vi "Write Map DVR 2.vi"(8 "error in (no error)":errorcluster, 10 "Map DVR":T1, 11 "Awesome! in":refnum<class "Awesome!.lvclass">) -> (0 "error out":errorcluster, 3 "Awesome! out":refnum<class "Awesome!.lvclass">)   [LabVIEW 2016, in "Awesome!.lvclass"]
uses:
  Awesome!.lvclass
  Common/Map DVR.ctl
  Common/Location Data.ctl
  Awesome!.lvclass/Awesome!.ctl
  Common/Common.lvlib
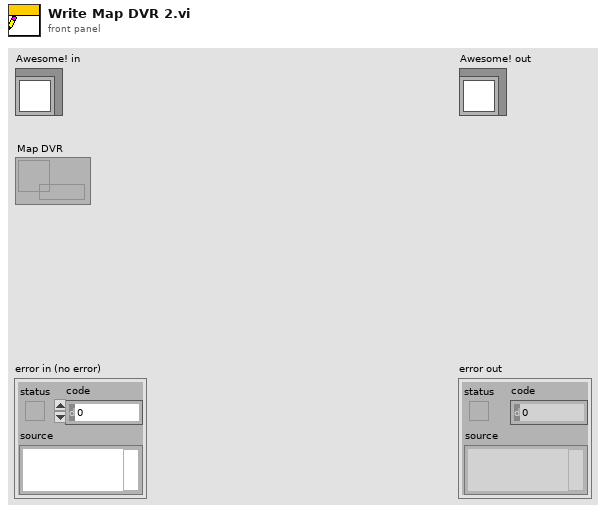
[diagram p1: front panel]
types:
  T1 = typedef "Common.lvlib/Map DVR.ctl" = refnum<data-value>
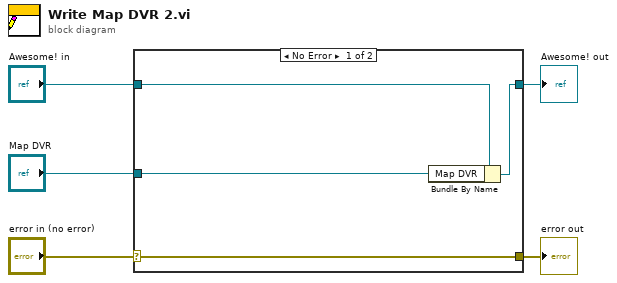
[diagram p0: block diagram]
diagram:
  n1 = case shown="No Error" "error in (no error)" {
    selector: "error in (no error)" -> [w9 w10]
    tunnel: [w9 w10] -> w4
    tunnel: [w7 w11] -> w2
    tunnel: "Awesome! in" -> [w8 w11]
    tunnel: "Map DVR" -> [w6 _]
    frame No Error {
      n2 = Bundle By Name(cluster=w8, "Map DVR"=w6) -> (w7:refnum<class "Awesome!.lvclass">)
    }
    frame Error {
    }
  }
  "error out" <- w4
  "Awesome! out" <- w2
